vi "RIO OK Control Loop.vi"   [LabVIEW 2015]
uses:
  <vilib>/Platform/TimedLoop/XDataNode/timing_clust.ctl
  <vilib>/Platform/TimedLoop/XDataNode/nitl_modes.ctl
  <vilib>/Platform/TimedLoop/XDataNode/wakeup.ctl
  Dashboard/SDashLEDs.ctl
  <vilib>/FPGAPlugInAG/sbRIO-9627/niLvFpga_Open_sbRIO-9627.vi
  Global Data.vi
  <vilib>/Utility/error.llb/Error Cluster From Error Code.vi
  <vilib>/rvi/errors/niLvFpgaAdjustHostInterfaceError.vi
  <vilib>/rvi/interface/nirviOpenFPGA/nirviOpenFPGA.xnode
  FPGA Bitfiles/Latest.lvbitx
  <vilib>/Platform/TimedLoop/XDataNode/XDataNode.xnode
  <vilib>/rvi/interface/nirviReadWriteControl/nirviReadWriteControl.xnode
  FPGA Typedef.ctl
  <vilib>/Platform/TimedLoop/XDataNode/XDNodeRunTimeDep.lvlib
  NiFpgaLv.dll
types:
  T1 = typedef "XDNodeRunTimeDep.lvlib/timing_clust.ctl" = cluster{"Expected End [f-1]":u64, "Actual End [f-1]":u64, "Finished Late? [f-1]":bool, "Expected End [i-1]":u64, "Actual End [i-1]":u64, "Finished Late? [i-1]":bool, "Expected Start [i]":u64, "Actual Start [i]":u64, "Expected Start [f]":u64, "Actual Start [f]":u64, "Source Name":string, "Structure Name":string, "Period":i64, "Deadline":i64, "Offset":i64, "Start":i64, "Priority":i32, "Timeout":i32, "Mode":T2, "Wakeup Reason":T3, "Error":errorcluster, "Source Type":string, "Secondary Source Type":string, "Global End Time":u64, "Global Start Time":u64, "Frame Duration":u64, "Iteration Duration":u64, "Assigned CPU":i32, "I/O Scan Engine Mode":u32}
  T2 = typedef "XDNodeRunTimeDep.lvlib/nitl_modes.ctl" = enum32{"No Change", "Process missed periods, maintain original phase", "Discard missed periods, maintain original phase", "Process missed periods, ignore original phase", "Discard missed periods, ignore original phase"}
  T3 = typedef "XDNodeRunTimeDep.lvlib/wakeup.ctl" = enum32{"Normal", "Aborted", "Asynchronous wakeup", "Timing source error", "Timed loop error", "Timeout"}
  T4 = typedef "SDashLEDs.ctl" = cluster{"bAMSLED":bool, "bUnsolderedED":bool, "bIMDLED":bool}
  T5 = typedef "Subsystem Status.ctl" = cluster{"eStatusSeverity":T6, "NValue":sgl, "CMessage":T7, "bNotOK":bool}
  T6 = typedef "Subsystem Status Severity.ctl" = enum16{"Okay", "Short Warning", "Long Warning", "Return to Pits", "Error", "Danger"}
  T7 = typedef "Subsystem Status Message.ctl" = enum16{"ControllerTemperature", "MotorTemperature", "BatteryTemperature", "BatteryLowVoltage", "LVBattery", "sbRIOTemperature", "Precharge", "BSPD", "IMD", "RemoteReturnToPits", "EStopInterrupted", "NoCellComms", "MCOverSpeed", "MCOverCurrent", "MCOverVoltage", "MCInverterOverTemp", "MCDirectionCommand", "MCInverterTimeout", "MCDesatFault", "MCHWOverCurrent", "MCUnderVoltage", "MCCommandMessageLost", "MotorOverTemp", "MCModAOverTemp", "MCModBOverTemp", "MCModCOverTemp", "MCPCBOverTemp", "MCGateDrv1OverTemp", "MCDateDrv2OverTemp", "MCCurrentSensorFault", "MCResolverNotConnected", "ShutdownLatchTripped", "UnknownBMS", "RemoteEmergency"}
  T8 = typedef "FPGA Typedef.ctl" = refnum<k20>
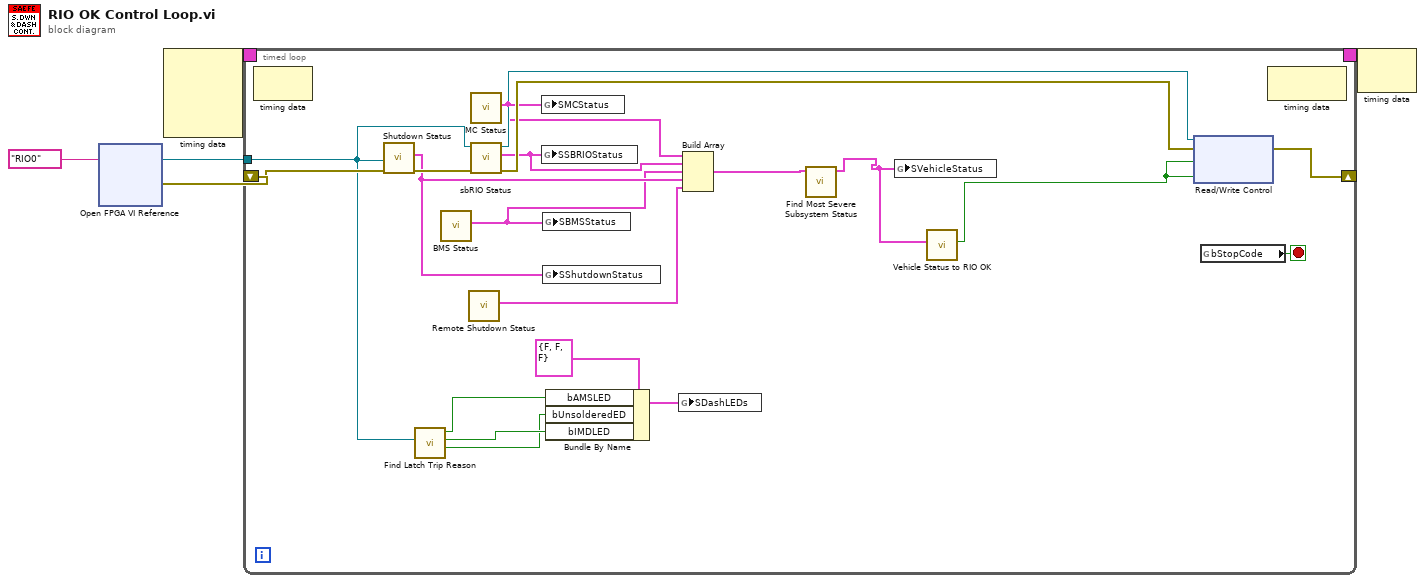
[diagram p0: block diagram]
diagram:
  n1 = xnode "Open FPGA VI Reference"("resource name"=tag "RIO0") -> ("FPGA VI Reference Out"=w1:refnum<k20>, "error out"=w5:errorcluster)  [unwired: 1 in]
  n2 = node-c288() -> (w4:T1)  [unwired: 4 in]
  n3 = timed-loop {
    shift-right: [w22] -> _
    shift-left: w5 -> [w25]
    timing: w4 -> [_]
    timing-out: [_] -> w3
    tunnel: w1 -> [w7]
    stop <- w21 stop-if-true
    n4 = node-c288() -> ()  [unwired: 1 in, 1 out]
    n5 = call "Shutdown Status.vi"("error in"=w25, "FPGA VI Reference In"=w7) -> ("error out"=w24:errorcluster, "Subsystem Status"=w17:T5)  [unwired: 7 in, 1 out]
    n6 = call "Find Latch Trip Reason.vi"("FPGA Interface"=w7) -> ("bBSPDDashLight"=w8:bool, "bIMDDashLight"=w9:bool, "bBMSDashLight"=w10:bool)  [unwired: 8 in]
    n7 = call "BMS Status.vi"() -> ("Subsystem Status"=w15:T5)  [unwired: 11 in]
    n8 = call "Remote Shutdown Status.vi"() -> ("Subsystem Status"=w16:T5)  [unwired: 11 in]
    n9 = call "MC Status.vi"() -> ("Subsystem Status"=w19:T5)  [unwired: 11 in]
    n10 = call "sbRIO Status.vi"("error in (no error)"=w24, "Refnum in"=w7) -> ("error out"=w23:errorcluster, "Subsystem Status"=w18:T5, "Refnum out"=w20:T8)  [unwired: 7 in]
    n11 = global write "Global Data.vi" "SMCStatus"(w19) -> ()
    n12 = global write "Global Data.vi" "SSBRIOStatus"(w18) -> ()
    n13 = global write "Global Data.vi" "SBMSStatus"(w15) -> ()
    n14 = global write "Global Data.vi" "SShutdownStatus"(w17) -> ()
    n15 = Bundle By Name(cluster=T4 {"bAMSLED"=FALSE, "bUnsolderedED"=FALSE, "bIMDLED"=FALSE} ("SDashLEDs"), "bAMSLED"=w10, "bUnsolderedED"=w8, "bIMDLED"=w9) -> (w11:T4)
    n16 = global write "Global Data.vi" "SDashLEDs"(w11) -> ()
    n17 = Build Array(w19, w18, w15, w17, w16) -> (w14:T5[])
    n18 = call "Find Most Severe Subsystem Status.vi"("Array"=w14) -> ("Subystem Status"=w13:T5)  [unwired: 10 in]
    n19 = global write "Global Data.vi" "SVehicleStatus"(w13) -> ()
    n20 = call "Vehicle Status to RIO OK.vi"("Vehicle Status"=w13) -> ("RIO OK"=w6:bool)  [unwired: 10 in]
    n21 = xnode "Read/Write Control"("FPGA VI Reference In"=w20, "error in"=w23, "bSBRIOOK1"=w6, "bSBRIOOK2"=w6) -> ("error out"=w22:errorcluster)  [unwired: 1 out]
    n22 = global read "Global Data.vi" "bStopCode"() -> (w21:bool)
    n23 = node-c288() -> ()  [unwired: 1 in, 1 out]
  }
  n24 = node-c288(w3) -> ()  [unwired: 1 out]
